vi "Move Inc.vi"(6 "Axis":string, 8 "error in (no error)":errorcluster, 9 "Speed":dbl format="%#_13g", 10 "Distance":dbl format="%#_13g", 11 "A3200 in":refnum<class "A3200.lvclass">) -> (0 "error out":errorcluster, 3 "A3200 out":refnum<class "A3200.lvclass">)   [LabVIEW 2016, in "A3200.lvclass"]
uses:
  A3200.lvclass
  Drivers/Aerotech A3200/Aerotech VIs.lvlib
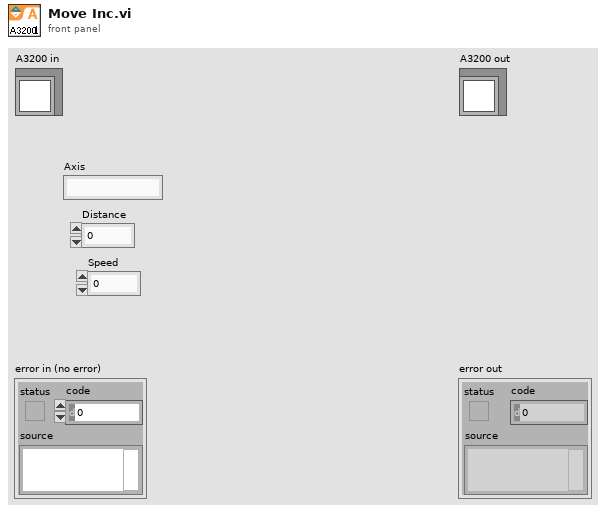
[diagram p1: front panel]
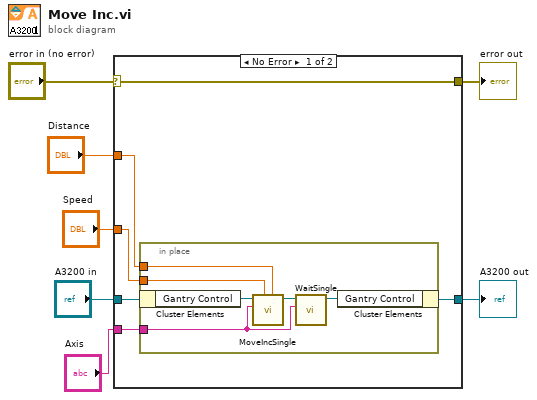
[diagram p0: block diagram]
diagram:
  n1 = case shown="No Error" "error in (no error)" {
    selector: "error in (no error)" -> [w11 w21]
    tunnel: "A3200 in" -> [w13 w20]
    tunnel: [w12 w20] -> w1
    tunnel: [w11 w21] -> w6
    tunnel: "Axis" -> [w10 _]
    tunnel: "Speed" -> [w9 _]
    tunnel: "Distance" -> [w8 _]
    frame No Error {
      n2 = in-place {
        in-place-border: w10 -> [w14]
        in-place-border: w9 -> [w18]
        in-place-border: w8 -> [w17]
        n3 = in-place-cluster #1(w13) -> ("Gantry Control"=w19:refnum<k24>)
        n4 = call "MoveIncSingle.vi"("distance"=w17, "speed"=w18, "axis name"=w14, "controller in"=w19) -> ("controller out"=w16:refnum<k24>)  [unwired: 6 in, 1 out]
        n5 = call "WaitSingle.vi"("axis name"=w14, "controller in"=w16) -> ("controller out"=w15:refnum<k24>)  [unwired: 7 in, 2 out]
        n6 = in-place-cluster #1("Gantry Control"=w15) -> (w12:refnum<class "A3200.lvclass">)
      }
    }
    frame Error {
    }
  }
  "error out" <- w6
  "A3200 out" <- w1
